vi "Secondary Xbox.vi"(10 "Secondary":T3, 11 "Dash Data In":T2={"Joy Stick"={"Primary"={"Buttons"={"A"=FALSE, "B"=FALSE, "X"=FALSE, "Y"=FALSE, "Left Bumper"=FALSE, "Right Bumper"=FALSE, "Back"=FALSE, "Start"=FALSE, "Left Thumbstick"=FALSE, "Right Thumbstick"=FALSE}, "Axes"={"Left Stick X "=0.0, "Left Stick Y"=0.0, "Triggers"=-0.0, "Right Stick X"=0.0, "Right Stick Y"=0.0, "D-Pad X"=0.0}}, "Secondary"={"Buttons"={"A"=FALSE, "B"=FALSE, "X"=FALSE, "Y"=FALSE, "Left Bumper"=FALSE, "Right Bumper"=FALSE, "Back"=FALSE, "Start"=FALSE, "Left Thumbstick"=FALSE, "Right Thumbstick"=FALSE}, "Axes"={"Left Stick X "=0.0, "Left Stick Y"=0.0, "Triggers"=0.0, "Right Stick X"=0.0, "Right Stick Y"=0.0, "D-Pad X"=0.0}}}, "Shooter"={"RPM Current"=0.0, "RPM Set"=0.0, "In Range?"=FALSE}, "Arm"={"Arm Current"=0.0, "Arm Set"=0.0, "At Position?"=FALSE, "Reset Encoder"=FALSE}, "Drive"={"Right"=0.0, "Left"=0.0}, "Climb State"=enum."Arm Attach", "Change Retical"=FALSE, "Solenoids"={"Robot Angle"=enum."Off", "Shooter Angle"=enum."Off", "Arm Lock"=enum."Off"}, "Shooter Speeds"=[]}) -> (3 "Dash Data Out 2":T2={"Joy Stick"={"Primary"={"Buttons"={"A"=FALSE, "B"=FALSE, "X"=FALSE, "Y"=FALSE, "Left Bumper"=FALSE, "Right Bumper"=FALSE, "Back"=FALSE, "Start"=FALSE, "Left Thumbstick"=FALSE, "Right Thumbstick"=FALSE}, "Axes"={"Left Stick X "=0.0, "Left Stick Y"=0.0, "Triggers"=-0.0, "Right Stick X"=0.0, "Right Stick Y"=0.0, "D-Pad X"=0.0}}, "Secondary"={"Buttons"={"A"=FALSE, "B"=FALSE, "X"=FALSE, "Y"=FALSE, "Left Bumper"=FALSE, "Right Bumper"=FALSE, "Back"=FALSE, "Start"=FALSE, "Left Thumbstick"=FALSE, "Right Thumbstick"=FALSE}, "Axes"={"Left Stick X "=0.0, "Left Stick Y"=0.0, "Triggers"=0.0, "Right Stick X"=0.0, "Right Stick Y"=0.0, "D-Pad X"=0.0}}}, "Shooter"={"RPM Current"=0.0, "RPM Set"=0.0, "In Range?"=FALSE}, "Arm"={"Arm Current"=0.0, "Arm Set"=0.0, "At Position?"=FALSE, "Reset Encoder"=FALSE}, "Drive"={"Right"=0.0, "Left"=0.0}, "Climb State"=enum."Arm Attach", "Change Retical"=FALSE, "Solenoids"={"Robot Angle"=enum."Off", "Shooter Angle"=enum."Off", "Arm Lock"=enum."Off"}, "Shooter Speeds"=[]})   [LabVIEW 2012]
uses:
  <vilib>/Rock Robotics/WPI/Solenoid/WPI_SolenoidValue.ctl
types:
  T1 = typedef "WPI_SolenoidValue.ctl" = enum16{"Off", "On", "Forward", "Reverse"}
  T2 = cluster{"Joy Stick":cluster{"Primary":cluster{"Buttons":cluster{"A":bool, "B":bool, "X":bool, "Y":bool, "Left Bumper":bool, "Right Bumper":bool, "Back":bool, "Start":bool, "Left Thumbstick":bool, "Right Thumbstick":bool}, "Axes":cluster{"Left Stick X ":dbl, "Left Stick Y":dbl, "Triggers":dbl, "Right Stick X":dbl, "Right Stick Y":dbl, "D-Pad X":dbl}}, "Secondary":cluster{"Buttons":cluster{"A":bool, "B":bool, "X":bool, "Y":bool, "Left Bumper":bool, "Right Bumper":bool, "Back":bool, "Start":bool, "Left Thumbstick":bool, "Right Thumbstick":bool}, "Axes":cluster{"Left Stick X ":dbl, "Left Stick Y":dbl, "Triggers":dbl, "Right Stick X":dbl, "Right Stick Y":dbl, "D-Pad X":dbl}}}, "Shooter":cluster{"RPM Current":dbl, "RPM Set":dbl, "In Range?":bool}, "Arm":cluster{"Arm Current":dbl, "Arm Set":dbl, "At Position?":bool, "Reset Encoder":bool}, "Drive":cluster{"Right":dbl, "Left":dbl}, "Climb State":enum16{"Arm Wait", "Arm Up", "Arm Down", "Arm Attach"}, "Change Retical":bool, "Solenoids":cluster{"Robot Angle":T1, "Shooter Angle":T1, "Arm Lock":T1}, "Shooter Speeds":dbl[]}
  T3 = cluster{"Buttons":cluster{"A":bool, "B":bool, "X":bool, "Y":bool, "Left Bumper":bool, "Right Bumper":bool, "Back":bool, "Start":bool, "Left Thumbstick":bool, "Right Thumbstick":bool}, "Axes":cluster{"Left Stick X ":dbl, "Left Stick Y":dbl, "Triggers":dbl, "Right Stick X":dbl, "Right Stick Y":dbl, "D-Pad X":dbl}}
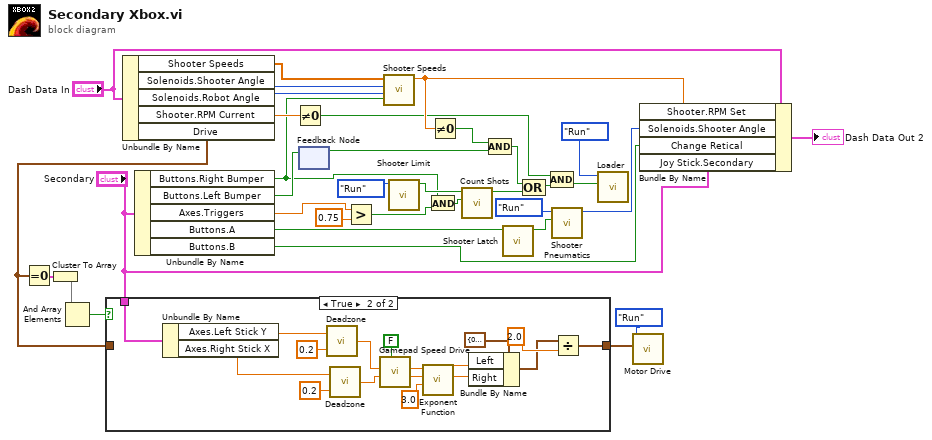
[diagram p0: block diagram]
diagram:
  n1 = Unbundle By Name("Dash Data In") -> ("Shooter Speeds"=w28:dbl[], "Solenoids.Shooter Angle"=w19:T1, "Solenoids.Robot Angle"=w21:T1, "Shooter.RPM Current"=w15:dbl, "Drive"=w7:cluster{"Right":dbl, "Left":dbl})
  n2 = Equal To 0?(x=w7) -> (x = 0?=w8:cluster{"Right":bool, "Left":bool})
  n3 = Cluster To Array(cluster=w8) -> (array=w6:bool[])
  n4 = And Array Elements(Boolean array=w6) -> (logical AND=w5:bool)
  n5 = case shown="True" w5 {
    tunnel: "Secondary" -> [_ w42]
    tunnel: [w36 w38] -> w9
    tunnel: w7 -> [w36 _]
    frame False {
    }
    frame True {
      n6 = Unbundle By Name(w42) -> ("Axes.Left Stick Y"=w41:dbl, "Axes.Right Stick X"=w40:dbl)
      n7 = call "Deadzone.vi"("Deadzone"=0.2, "Input"=w41) -> ("Output"=w49:dbl)
      n8 = call "Deadzone.vi"("Deadzone"=0.2, "Input"=w40) -> ("Output"=w47:dbl)
      n9 = call "Gamepad Speed Drive.vi"("Quick Turn"=FALSE, "Turn"=w47, "Speed"=w49) -> ("Right Output"=w52:dbl, "Left Output"=w53:dbl)  [unwired: 7 in]
      n10 = call "Exponent Function.vi"("Exponent"=3.0, "Left In"=w52, "Right In"=w53) -> ("Right Out"=w44:dbl, "Left Out"=w45:dbl)  [unwired: 7 in]
      n11 = Bundle By Name(cluster=cluster{"Right":dbl, "Left":dbl} {"Right"=0.0, "Left"=0.0} ("Motor"), "Left"=w45, "Right"=w44) -> (w39:cluster{"Right":dbl, "Left":dbl})
      n12 = Divide(x=w39, y=2.0) -> (x/y=w38:cluster{"Right":dbl, "Left":dbl})
    }
  }
  n13 = Unbundle By Name("Secondary") -> ("Buttons.Right Bumper"=w1:bool, "Buttons.Left Bumper"=w22:bool, "Axes.Triggers"=w17:dbl, "Buttons.A"=w35:bool, "Buttons.B"=w18:bool)
  n14 = Not Equal To 0?(x=w15) -> (x != 0?=w14:bool)
  n15 = feedback #1() -> (w26:bool)  [unwired: 1 in]
  n16 = feedback-in #1(w22) -> ()
  n17 = Greater?(x=w17, y=0.75) -> (0:w4:bool)
  n18 = call "Shooter Speeds.vi"("Right Bumper"=w1, "Robot Angle"=w21, "Shooter Angle"=w19, "Shooter Speeds"=w28) -> ("f"=w20:dbl)  [unwired: 7 in]
  n19 = call "Shooter Limit.vi"("Enum"=enum16{"Start", "Run", "End"}."Run") -> ("Value"=w23:bool)  [unwired: 10 in]
  n20 = And(x=w1, y=w4) -> (x .and. y?=w3:bool)
  n21 = Not Equal To 0?(x=w20) -> (x != 0?=w2:bool)
  n22 = call "Count Shots.vi"("Boolean in"=w3, "Value"=w23) -> ("Boolean out"=w24:bool)  [unwired: 9 in]
  n23 = Compound Arithmetic op=AND(w2, w26) -> (w16:bool)
  n24 = call "Shooter Latch.vi"("Input"=w35) -> ("Latched"=w34:bool)  [unwired: 10 in]
  n25 = Compound Arithmetic op=OR(w16, w24) -> (w12:bool)
  n26 = Compound Arithmetic op=AND(w14, w12) -> (w13:bool)
  n27 = call "Shooter Pneumatics.vi"("Boolean"=w34, "Enum"=enum16{"Start", "Run", "End"}."Run") -> ("Shooter Angle"=w31:T1)  [unwired: 9 in]
  n28 = call "Loader.vi"("Enum"=enum16{"Start", "Run", "End"}."Run", "Run"=w13) -> ()  [unwired: 9 in]
  n29 = call "Motor Drive.vi"("Motor"=w9, "Enum"=enum16{"Start", "Run", "End"}."Run") -> ()  [unwired: 10 in]
  n30 = Bundle By Name(cluster="Dash Data In", "Shooter.RPM Set"=w20, "Solenoids.Shooter Angle"=w31, "Change Retical"=w18, "Joy Stick.Secondary"="Secondary") -> (→"Dash Data Out 2":T2)
